vi "get VTK num Points.vi"(8 "error in (no error)":errorcluster) -> (0 "error out":errorcluster, 3 "function return":i32)   [LabVIEW 2019, in "libConvectionDiffusionWrapper.lvlib"]
doc: "int getVTK_numPoints();"
uses:
  libConvectionDiffusionWrapper.lvlib
  libConvectionDiffusionWrapper.so
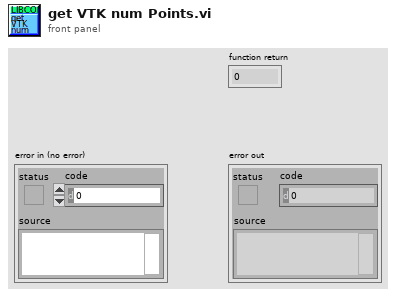
[diagram p1: front panel]
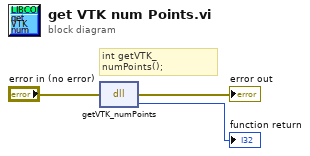
[diagram p0: block diagram]
diagram:
  # "int getVTK_numPoints();"
  n1 = dll-call lib="home/paul/Schreibtisch/Convection_diffusion/LabView/lib/libConvectionDiffusionWrapper/libConvectionDiffusionWrapper.*" fn="getVTK_numPoints"(error in="error in (no error)") -> (error out=→"error out":errorcluster, →"function return":i32)  [unwired: 2 in, 1 out]
